vi "RSZVB Set Color Scheme.vi"(8 "error in (no error)":errorcluster {"code" format="%.0x"}, 10 "Color Scheme (0: Dark Background)":i32(ring) items=["Dark Background", "Light Background", "B&W Line Styles", "B&W Solid"], 11 "VISA session":refnum<visa-resource-name>) -> (0 "error out":errorcluster {"code" format="%.0x"}, 3 "dup VISA session":refnum<visa-resource-name>)   [LabVIEW 2011]
doc: "This VI selects the color scheme for all diagram areas in the active setup.\n\nRemote-control command(s):\nSYSTem:DISPlay:COLor DBACkground | LBACkground | BWLStyles | BWSolid"
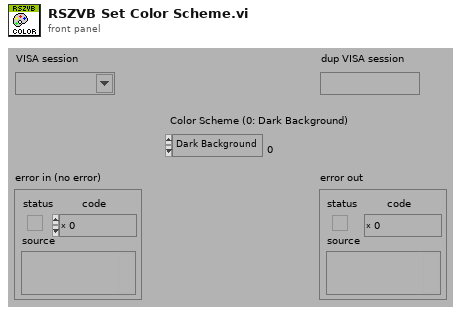
[diagram p1: front panel]
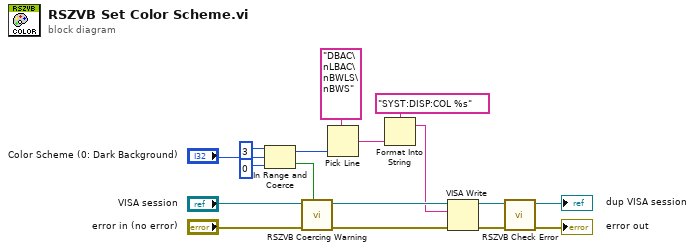
[diagram p0: block diagram]
diagram:
  n1 = In Range and Coerce(upper limit=3, x="Color Scheme (0: Dark Background)", lower limit=0) -> (coerced(x)=w8:i32, In Range?=w1:bool)
  n2 = call "RSZVB Coercing Warning.vi"("In Range?"=w1, "error in (no error)"="error in (no error)", "VISA session"="VISA session") -> ("error out"=w13:errorcluster, "dup VISA session"=w14:refnum<visa-resource-name>)  [unwired: 7 in]
  n3 = Pick Line(multi-line string="DBAC\nLBAC\nBWLS\nBWS", line index=w8) -> (output string=w7:string)  [unwired: 1 in]
  n4 = Format Into String(format string="SYST:DISP:COL %s", w7) -> (resulting string=w10:string)  [unwired: 2 in, 1 out]
  n5 = VISA Write(VISA resource name=w14, write buffer=w10, error in (no error)=w13) -> (VISA resource name out=w11:refnum<visa-resource-name>, error out=w12:errorcluster)  [unwired: 1 out]
  n6 = call "RSZVB Check Error.vi"("error in (no error)"=w12, "VISA session"=w11) -> ("error out"=→"error out":errorcluster, "dup VISA session"=→"dup VISA session":refnum<visa-resource-name>)  [unwired: 8 in]
